vi "Read Run and enable.vi"(8 "error in (no error)":errorcluster, 11 "Master CR in":refnum<class "WebSocket Client CR.lvclass">) -> (0 "error out":errorcluster, 2 "Enable and Run":bool, 3 "Master CR out":refnum<class "WebSocket Client CR.lvclass">)   [LabVIEW 2021, in "WebSockets.lvlib" / "WebSocket Client CR.lvclass"]
uses:
  WebSocket Client CR.lvclass
  WebSocket Client CR.lvclass/WebSocket Client CR.ctl
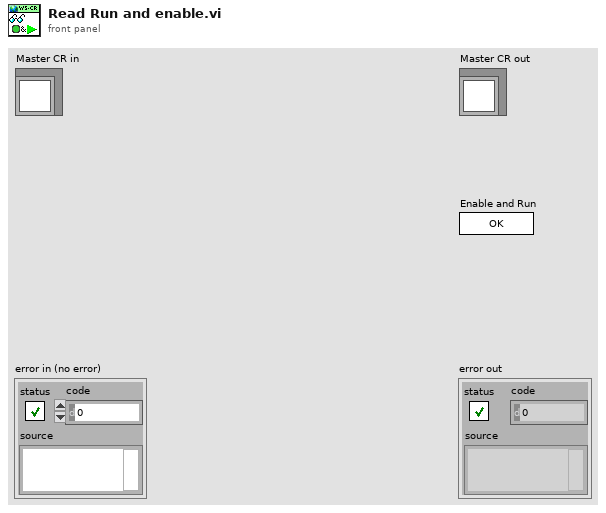
[diagram p1: front panel]
types:
  T1 = typedef "WebSockets.lvlib/WebSocket Client CR.lvclass/Master CR state.ctl" = cluster{"state":T2, "enable":bool, "write enable":bool, "connect":bool, "errors":i32, "Run":bool, "Write":bool, "Stop":bool}
  T2 = typedef "WebSockets.lvlib/WebSocket Client CR.lvclass/CR_Core_State.ctl" = enum8{"initialization", "redefine", "standby", "ping", "connect", "wait to reconnect", "wait to reset timeout", "configure", "requests", "close connection", "stop"}
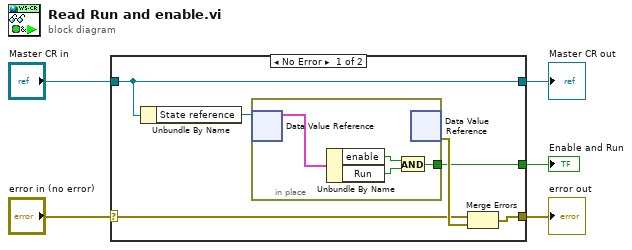
[diagram p0: block diagram]
diagram:
  n1 = case shown="No Error" "error in (no error)" {
    selector: "error in (no error)" -> [w8 w17]
    tunnel: [w9 w17] -> w4
    tunnel: "Master CR in" -> [w7 w16]
    tunnel: [w7 w16] -> w2
    tunnel: [w6 _] -> w1
    frame No Error {
      n2 = Unbundle By Name(w7) -> ("State reference"=w11:refnum<data-value>)
      n3 = in-place {
        in-place-border: [w12] -> w6
        n4 = in-place-dvr #1(w11) -> (w15:T1)  [unwired: 1 out]
        n5 = Unbundle By Name(w15) -> ("enable"=w13:bool, "Run"=w14:bool)
        n6 = And(x=w13, y=w14) -> (x .and. y?=w12:bool)
        n7 = in-place-dvr #1() -> (w10:errorcluster)  [unwired: 1 in, 1 out]
      }
      n8 = Merge Errors(w8, w10) -> (w9:errorcluster)
    }
    frame Error {
    }
  }
  "error out" <- w4
  "Master CR out" <- w2
  "Enable and Run" <- w1
